vi "Fan State Trace.vi"(4 "error in (no error)":errorcluster, 6 "Launch Order":i32, 7 "Fan State":enum16{"Off", "On"}(ring)) -> (0 "error out":errorcluster)   [LabVIEW 2020, in "Startup Processes.lvlib"]
uses:
  Startup Processes.lvlib
  toolbox/Debugging/Debugging.lvlib
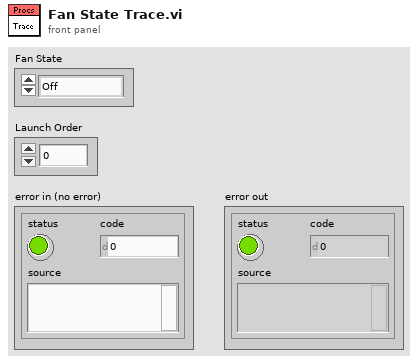
[diagram p1: front panel]
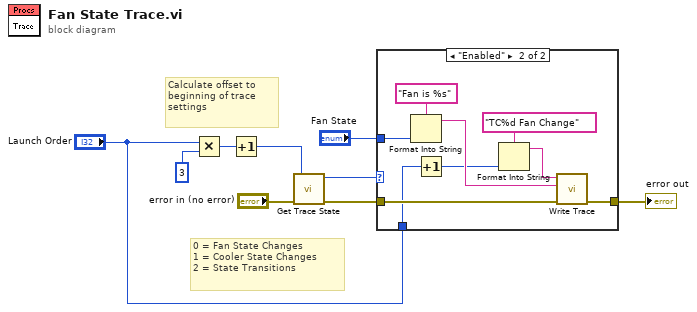
[diagram p0: block diagram]
diagram:
  # "0 = Fan State Changes\n1 = Cooler State Changes\n2 = State Transitions"
  # "Calculate offset to beginning of trace settings"
  n1 = Multiply(x="Launch Order", y=3) -> (x*y=w8:i32)
  n2 = Increment(x=w8) -> (x+1=w7:i32)
  n3 = call "Get Trace State.vi"("Error In"="error in (no error)", "Trace Point Index"=w7) -> ("Error Out"=w5:errorcluster, "Trace Point State"=w4:enum16{"Disabled", "Enabled"})  [unwired: 4 in]
  n4 = case shown="\"Enabled\"" w4 {
    tunnel: w5 -> [w10 w19]
    tunnel: [w10 w18] -> w2
    tunnel: "Fan State" -> [_ w17]
    tunnel: "Launch Order" -> [_ w11]
    frame "Disabled" {
    }
    frame "Enabled" {
      n5 = Format Into String(format string="Fan is %s", w17) -> (resulting string=w16:string)  [unwired: 2 in, 1 out]
      n6 = Increment(x=w11) -> (x+1=w12:i32)
      n7 = Format Into String(format string="TC%d Fan Change" ("Trace Point Name"), w12) -> (resulting string=w13:string)  [unwired: 2 in, 1 out]
      n8 = call "Write Trace.vi"("Error In"=w19, "Trace Data"=w16, "Trace Point Name"=w13) -> ("Error Out"=w18:errorcluster)  [unwired: 4 in]
    }
  }
  "error out" <- w2
